vi "Read VariablesStatus.vi"(8 "error in (no error)":errorcluster, 11 "CoolerControler in":refnum<class "CoolerControler.lvclass">) -> (0 "error out":errorcluster, 2 "VariablesStatus":T1, 3 "CoolerControler out":refnum<class "CoolerControler.lvclass">)   [LabVIEW 2016, in "CoolerControler.lvclass"]
uses:
  CoolerControler.lvclass
  typedefs/ControlVariablesStatus.ctl
  CoolerControler.lvclass/CoolerControler.ctl
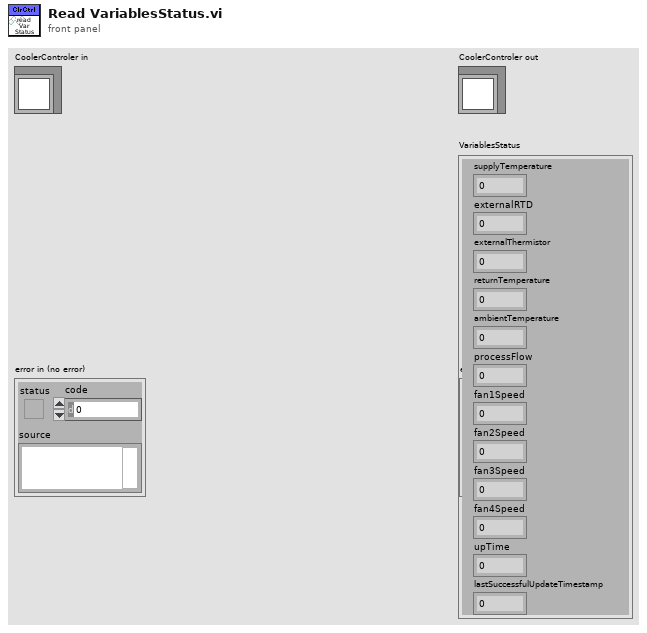
[diagram p1: front panel]
types:
  T1 = typedef "ControlVariablesStatus.ctl" = cluster{"supplyTemperature":dbl, "externalRTD":dbl, "externalThermistor":dbl, "returnTemperature":dbl, "ambientTemperature":dbl, "processFlow":dbl, "fan1Speed":dbl, "fan2Speed":dbl, "fan3Speed":dbl, "fan4Speed":dbl, "upTime":dbl, "lastSuccessfulUpdateTimestamp":dbl}
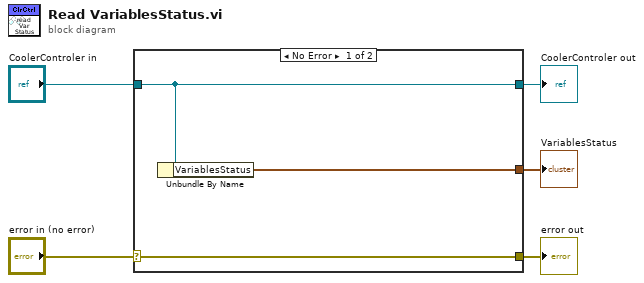
[diagram p0: block diagram]
diagram:
  n1 = case shown="No Error" "error in (no error)" {
    selector: "error in (no error)" -> [w8 w9]
    tunnel: [w8 w9] -> w4
    tunnel: [w7 w10] -> w2
    tunnel: "CoolerControler in" -> [w7 w10]
    tunnel: [w6 _] -> w1
    frame No Error {
      n2 = Unbundle By Name(w7) -> ("VariablesStatus"=w6:T1)
    }
    frame Error {
    }
  }
  "error out" <- w4
  "CoolerControler out" <- w2
  "VariablesStatus" <- w1
